vi "CLSUIP_GrowRightDirection.vi"(2 "Multiplication Factor":i32, 3 "lower":i16, 4 "higher":i16, 5 "point":i32) -> (0 "new lower":i16, 1 "new higher":i16)   [LabVIEW 2021, in "MemberVICreation.lvlib" / "VIRetooler.lvclass"]
uses:
  <resource>/Framework/Providers/LVClassLibrary/NewAccessors/VIRetooler/VIRetooler.lvclass
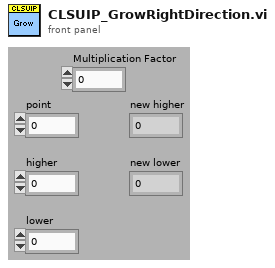
[diagram p1: front panel]
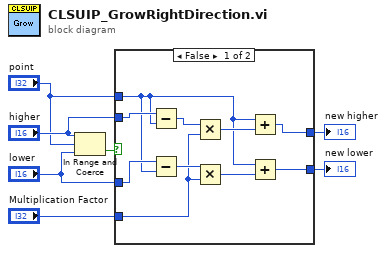
[diagram p0: block diagram]
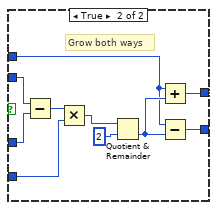
[diagram p2: hidden frame]
diagram:
  n1 = In Range and Coerce(upper limit="higher", x="point", lower limit="lower") -> (In Range?=w5:bool)  [unwired: 1 out]
  n2 = case shown="False" w5 {
    tunnel: "higher" -> [w17 w23]
    tunnel: "lower" -> [w16 w21]
    tunnel: "Multiplication Factor" -> [w13 w26]
    tunnel: [w9 w22] -> w3
    tunnel: [w8 w19] -> w2
    tunnel: "point" -> [w10 w18]
    frame False {
      n3 = Subtract(x=w17, y=w10) -> (x-y=w15:i32)
      n4 = Subtract(x=w16, y=w10) -> (x-y=w14:i32)
      n5 = Multiply(x=w15, y=w13) -> (x*y=w12:i32)
      n6 = Multiply(x=w14, y=w13) -> (x*y=w11:i32)
      n7 = Add(x=w10, y=w12) -> (x+y=w9:i32)
      n8 = Add(x=w10, y=w11) -> (x+y=w8:i32)
    }
    frame True {
      # "Grow both ways"
      n9 = Subtract(x=w23, y=w21) -> (x-y=w27:i16)
      n10 = Multiply(x=w27, y=w26) -> (x*y=w25:i32)
      n11 = Quotient & Remainder(x=w25, y=2) -> (floor(x/y)=w20:i32)  [unwired: 1 out]
      n12 = Add(x=w18, y=w20) -> (x+y=w22:i32)
      n13 = Subtract(x=w18, y=w20) -> (x-y=w19:i32)
    }
  }
  "new lower" <- w2
  "new higher" <- w3
